vi "getUserEvent.vi"(8 "error in (no error)":errorcluster, 11 "Observer in":refnum<class "Observer.lvclass">) -> (0 "error out":errorcluster, 2 "UserEvent":refnum<user-event>, 3 "Observer out":refnum<class "Observer.lvclass">)   [LabVIEW 2020, in "Observer.lvclass"]
uses:
  Observer.lvclass
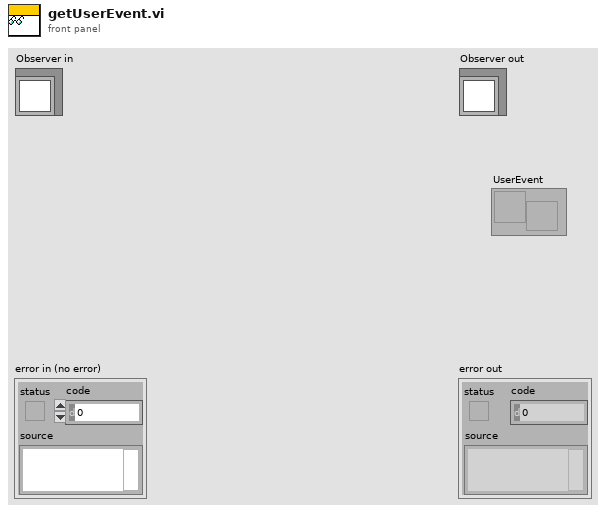
[diagram p1: front panel]
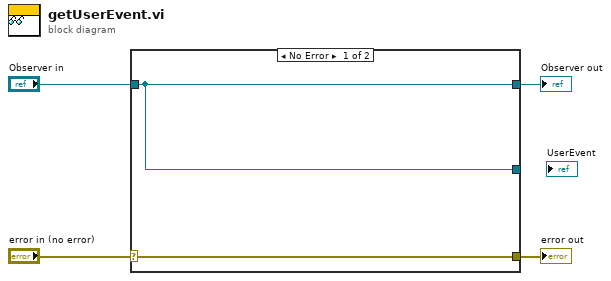
[diagram p0: block diagram]
diagram:
  n1 = case shown="No Error" "error in (no error)" {
    selector: "error in (no error)" -> [w6 w7]
    tunnel: [w6 w7] -> w3
    tunnel: [w5 w8] -> w1
    tunnel: "Observer in" -> [w5 w8]
    tunnel: [w5 _] -> _
    frame No Error {
    }
    frame Error {
    }
  }
  "error out" <- w3
  "Observer out" <- w1
